vi "Book_Find.vi"(8 "error in (no error)":errorcluster, 11 "generated coordinates":cluster{"X":sgl, "Y":sgl}) -> (0 "error out":errorcluster, 1 "Found?":bool, 2 "Detector Index":i32, 3 "Nearest Detector":string)   [LabVIEW 2020]
doc: "Identifies the detector that can detect the book. Displays \"NOT FOUND\" if book is not found within radius of any detector."
uses:
  <vilib>/vision/NI_Vision_Development_Module.lvlib
panel:
  out "Filtered_Array":dbl[](array[numeric])
  out "Radius Array":dbl[](array[numeric])
  out "Difference Array":dbl[](array[numeric])
  out "Distance Array":sgl[](array[numeric])
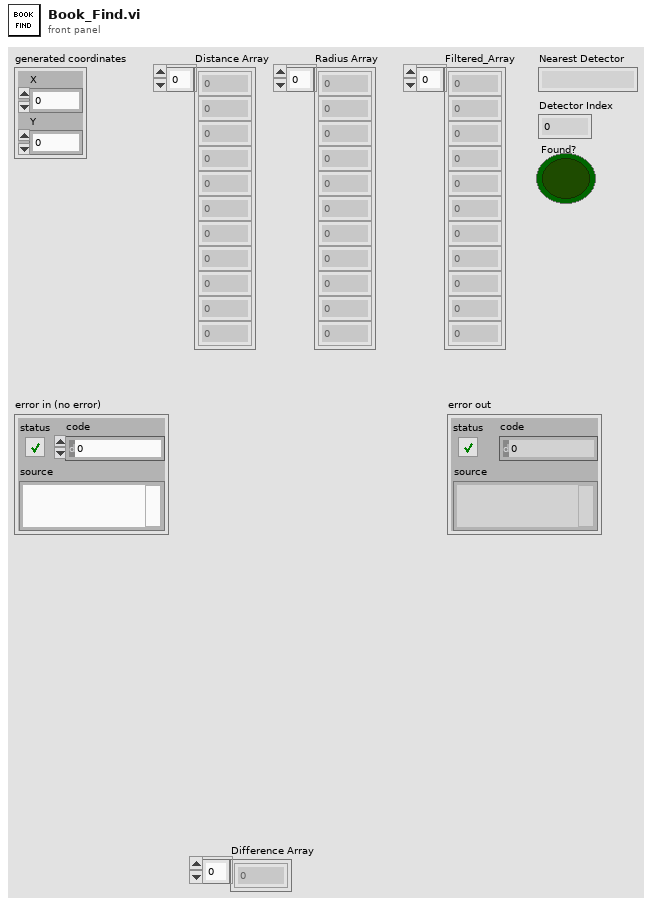
[diagram p1: front panel]
types:
  T1 = typedef "Image_Cluster.ctl" = cluster{"Detector_info":cluster{"No. of detectors":dbl, "Detector_Array":string[][], "Detector_Array_Numeric":dbl[][]}, "Corner_info":cluster{"Corner_Array":dbl[][]}, "ROI":cluster{"Corners":cluster{"Global Rectangle":i32[], "Contours":cluster{"ID":enum32{"External", "Internal"}, "Type":u32, "Coordinates":i32[]}[]}[], "Detectors":cluster{"Global Rectangle":i32[], "Contours":cluster{"ID":enum32{"External", "Internal"}, "Type":u32, "Coordinates":i32[]}[]}[]}, "Shape_Detect":cluster{"Match_score":dbl, "Curve Parameters":T2, "Match Options":T3, "Circle Descriptor":cluster{"Min Radius":dbl, "Max Radius":dbl}}, "Path":cluster{"Config":path, "Map":path}, "Map":cluster{"X_resolution":i32, "Y_resolution":i32, "Image":T5}}
  T2 = typedef "IMAQ Curve Parameters.ctl" = cluster{"Extraction Mode":u32, "Edge Threshold":i32, "Edge Filter Size":u32, "Min Length":i32, "Row Search Step Size":i32, "Col Search Step Size":i32, "Max Endpoint Gap":i32, "Closed":bool, "Subpixel":bool}
  T3 = typedef "ShapeDetectionMatchOptions.ctl" = cluster{"Rotation":bool, "Scale":bool, "Occlusion":bool, "Range Settings":T4[]}
  T4 = typedef "IMAQ Match Range Setting.ctl" = cluster{"Match Constraints":u32, "Min":dbl, "Max":dbl}
  T5 = typedef "IMAQ Image.ctl" = refnum<image>
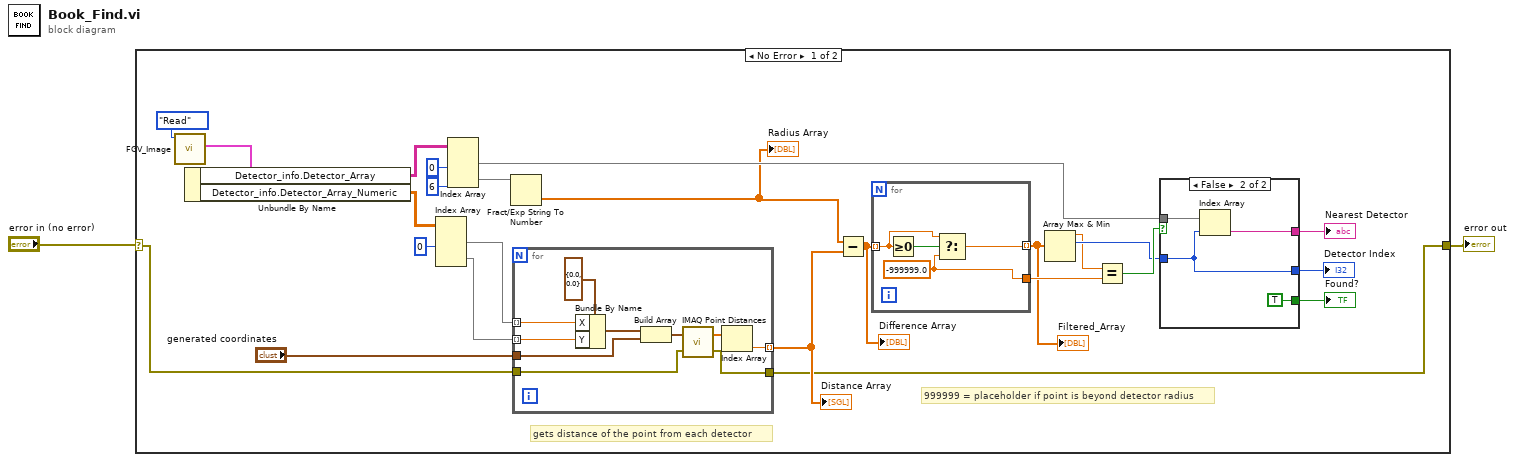
[diagram p0: block diagram]
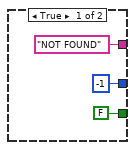
[diagram p2: hidden frame]
diagram:
  n1 = case shown="No Error" "error in (no error)" {
    selector: "error in (no error)" -> [w7 w49]
    tunnel: [w6 w49] -> w1
    frame No Error {
      # "gets distance of the point from each detector"
      # "999999 = placeholder if point is beyond detector radius"
      n2 = call "FGV_Image.vi"("Action"=enum16{"Read", "Write", ""}."Read") -> ("Image_Cluster_out"=w10:T1)  [unwired: 10 in]
      n3 = Unbundle By Name(w10) -> ("Detector_info.Detector_Array"=w16:string[][], "Detector_info.Detector_Array_Numeric"=w11:dbl[][])
      n4 = Index Array(array=w11, index (col) #1=0 ("disabled index (col)")) -> (element #1=w13:dbl[], element #2=w14:dbl[])  [unwired: 3 in]
      n5 = Index Array(array=w16, index (col) #1=0 ("disabled index (col)"), index (col) #2=6 ("index (col)")) -> (element #1=w23:string[], element #2=w22:string[])  [unwired: 2 in]
      n6 = Fract/Exp String To Number(string=w22) -> (number=w18:dbl[])  [unwired: 3 in, 1 out]
      "Radius Array" <- w18
      n7 = for {
        tunnel: w13 -> [w47] mode=indexing
        tunnel: w14 -> [w46] mode=indexing
        tunnel: "generated coordinates" -> [w44]
        tunnel: [w41] -> w19 mode=indexing
        tunnel: w7 -> [w40]
        tunnel: [w39] -> w6
        n8 = Bundle By Name(cluster=cluster{"X":sgl, "Y":sgl} {"X"=0.0, "Y"=0.0}, "X"=w47, "Y"=w46) -> (w45:cluster{"X":sgl, "Y":sgl})
        n9 = Build Array(w45, w44) -> (w43:cluster{"X":sgl, "Y":sgl}[])
        n10 = call "IMAQ Point Distances"("Points"=w43, "error in (no error)"=w40) -> ("Distances"=w42:sgl[], "error out"=w39:errorcluster)  [unwired: 3 in]
        n11 = Index Array(array=w42) -> (element=w41:sgl)  [unwired: 1 in]
      }
      "Distance Array" <- w19
      n12 = Subtract(x=w18, y=w19) -> (x-y=w24:dbl[])
      "Difference Array" <- w24
      n13 = for {
        tunnel: w24 -> [w36] mode=indexing
        tunnel: [w37] -> w20 mode=indexing
        tunnel: [w35] -> w26
        w35 = -999999.0 ("f")
        n14 = Greater Or Equal To 0?(x=w36) -> (x >= 0?=w38:bool)
        n15 = Select(t=w36, s=w38, f=w35) -> (s? t:f=w37:dbl)
      }
      "Filtered_Array" <- w20
      n16 = Array Max & Min(array=w20) -> (max value=w3:dbl, max index (indices)=w4:i32)  [unwired: 2 out]
      n17 = Equal?(x=w3, y=w26) -> (x = y?=w27:bool)
      n18 = case shown="False" w27 {
        tunnel: w23 -> [_ w34]
        tunnel: w4 -> [_ w32]
        tunnel: ["NOT FOUND" ("String") w33] -> w25
        tunnel: [-1 w32] -> w8
        tunnel: [FALSE TRUE] -> w5
        frame True {
        }
        frame False {
          n19 = Index Array(array=w34, index=w32) -> (element=w33:string)
        }
      }
      "Nearest Detector" <- w25
      "Detector Index" <- w8
      "Found?" <- w5
    }
    frame Error {
    }
  }
  "error out" <- w1
